vi "Large_LUT_Mode_Slave_flash_.vi"(8 "error in (no error)":errorcluster, 9 "SequenceId":u32, 10 "DeviceIdPtr in":u32, 11 "LUT":i32[](array[numeric])) -> (0 "error out":errorcluster, 1 "SequenceId Out":u32, 2 "DeviceId Out":u32)   [LabVIEW 2020]
panel:
  out "Array 2":i32[][](array[numeric])
  out "Array":i32[](array[numeric])
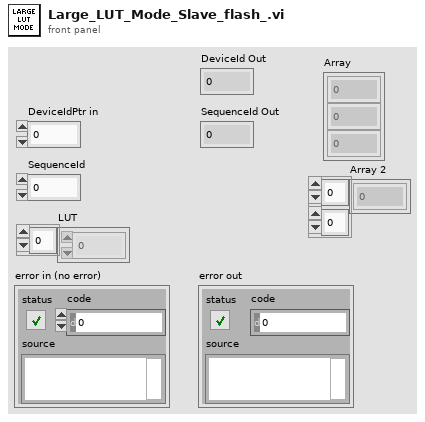
[diagram p1: front panel]
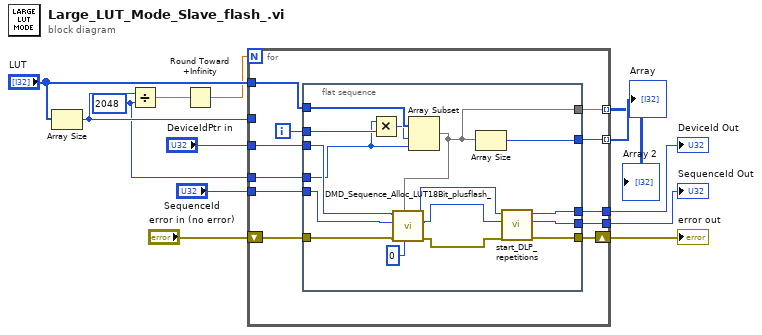
[diagram p0: block diagram]
diagram:
  w2 = 2048 ("y")
  n1 = Array Size(array="LUT") -> (size(s)=w13:i32)
  n2 = Divide(x=w13, y=w2) -> (x/y=w10:dbl)
  n3 = Round Toward +Infinity(x=w10) -> (ceil(x): smallest int >= x=w11:dbl)
  n4 = for {
    N: w11 -> [_]
    tunnel: [w24] -> w4
    tunnel: [w23] -> w5
    tunnel: "DeviceIdPtr in" -> [w21]
    tunnel: "SequenceId" -> [w20]
    tunnel: "LUT" -> [w18]
    shift-right: [w22] -> w6
    shift-left: "error in (no error)" -> [w19]
    tunnel: w13 -> [_]
    tunnel: [w16] -> w3 mode=indexing
    tunnel: w2 -> [w15]
    tunnel: [w14] -> w1 mode=indexing
    i -> [w17]
    n5 = flat-sequence {
      tunnel: [w38] -> w22
      tunnel: [w39] -> w23
      tunnel: [w40] -> w24
      tunnel: w17 -> [w35]
      tunnel: w18 -> [w37]
      tunnel: w19 -> [w32]
      tunnel: w20 -> [w33]
      tunnel: w21 -> [w34]
      tunnel: [w27] -> w16
      tunnel: w15 -> [w26]
      tunnel: [w25] -> w14
      frame #0 {
        n6 = Multiply(x=w26, y=w35) -> (x*y=w36:i32)
        n7 = Array Subset(array=w37, index=w36, length=w26) -> (w25:i32[])
        n8 = call "DMD_Sequence_Alloc_LUT18Bit_plusflash_.vi"("nOffset"=0, "LUT incl. diff"=w25, "error in (no error)"=w32, "SequenceId"=w33, "DeviceId"=w34) -> ("error out"=w31:errorcluster, "SequenceId Out"=w30:u32, "DeviceId Out"=w29:u32)  [unwired: 4 in]
        n9 = Array Size(array=w25) -> (size(s)=w27:i32)
        n10 = call "start_DLP_repetitions.vi"("error in (no error)"=w31, "SequenceId"=w30, "DeviceId"=w29) -> ("error out"=w38:errorcluster, "SequenceId Out"=w39:u32, "DeviceId Out"=w40:u32)  [unwired: 6 in]
      }
    }
  }
  "error out" <- w6
  "SequenceId Out" <- w5
  "DeviceId Out" <- w4
  "Array" <- w3
  "Array 2" <- w1
